vi "online_nonlinear_calibration_save(subVI).vi"(8 "error in (no error)":errorcluster, 9 "Grid Descriptor":cluster{"X Step":sgl, "Y Step":sgl, "Unit":T2}={"X Step"=10.0, "Y Step"=10.0, "Unit"=enum."Millimeter"}, 10 "Image Type":T3 items=["Grayscale (U8)", "Grayscale (I16)", "Grayscale (SGL)", "Complex (CSG)", "RGB (U32)", "HSL (U32)", "RGB (U64)", "Grayscale (U16)"], 11 "Session In":T4="cam0") -> (0 "error out":errorcluster={"status"=TRUE, "code"=-1074396116, "source"="IMAQ CalibrationTargetToPoints\n  "}, 2 "Calibration Axis Info":T5={"Origin Pixel"={"X"=0.0, "Y"=0.0}, "Angle Relative to Horizontal (deg)"=0.0, "X Axis Pixel"={"X"=0.0, "Y"=0.0}, "Axis Reference"=1} {"X Axis Pixel"."Y" format="%.2f"; "X Axis Pixel"."X" format="%.2f"; "Axis Reference" items=["Direct", "Indirect"]; "Angle Relative to Horizontal (deg)" format="%.2f"; "Origin Pixel"."Y" format="%.2f"; "Origin Pixel"."X" format="%.2f"}, 3 "Calibration Template Image Out":T1)   [LabVIEW 2020]
uses:
  <vilib>/vision/Calibration.llb/Error Statistics.ctl
  <vilib>/userDefined/High Color/IMAQdx.ctl
  <vilib>/vision/Image Controls.llb/IMAQ Image.ctl
  <vilib>/vision/Calibration.llb/Distortion Model.ctl
  <vilib>/vision/Calibration.llb/Distortion Model Types.ctl
  <vilib>/vision/NI_Vision_Development_Module.lvlib
panel:
  out "Grey scale image":T1(plugin-control)
  in  "File Path":path=path "D:/desktop/sistemi di visione/foto/calib_info.png"
  out "Error Statistics":T6
  out "Error Map":sgl[][](array[numeric]) format="%.2f"
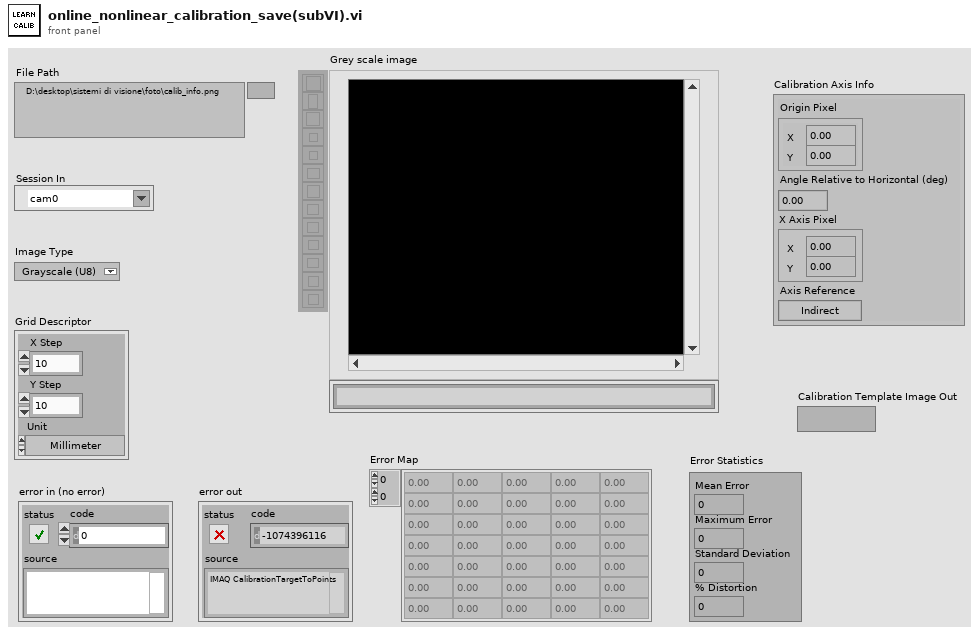
[diagram p1: front panel]
types:
  T1 = typedef "IMAQ Image.ctl" = refnum<image>
  T2 = typedef "Image Unit" = enum32{"Undefined", "Angström", "Micrometer", "Millimeter", "Centimeter", "Meter", "Kilometer", "Microinch", "Inch", "Feet", "Nautical miles", "Standard miles", "Steps"}
  T3 = typedef "Image Type" = u32
  T4 = typedef "IMAQdx.ctl" = refnum<k21>
  T5 = cluster{"Origin Pixel":cluster{"X":sgl, "Y":sgl}, "Angle Relative to Horizontal (deg)":sgl, "X Axis Pixel":cluster{"X":sgl, "Y":sgl}, "Axis Reference":u32}
  T6 = typedef "Error Statistics.ctl" = cluster{"Mean Error":dbl, "Maximum Error":dbl, "Standard Deviation":dbl, "% Distortion":dbl}
  T7 = cluster{"Origin Pixel":cluster{"X":sgl, "Y":sgl}, "Angle Relative to Horizontal (deg)":sgl, "Axis Reference":u32}
  T8 = typedef "Distortion Model.ctl" = cluster{"Distortion Model":T9, "Polynomial Model Setup":cluster{"Radial Coefficient":u32, "Tangential Coefficients ":bool}}
  T9 = typedef "Distortion Model Types.ctl" = i32
  T10 = typedef "Particle Parameters" = i32
  T11 = cluster{"Measurement Parameter":T10, "Range Lower Value":dbl, "Range Upper Value":dbl, "Range":bool, "Measurement Type":bool}[]
  T12 = cluster{"Desired Font (Application)":enum16{"User-specified Font", "Application Font", "System Font", "Dialog Font"}, "[User-specified Font]":cluster{"Font Name":string, "Size":i16, "Strikeout?":bool, "Italic?":bool, "Underline?":bool, "Outline?":bool, "Shadow?":bool, "Bold?":bool, "Rotation Angle":dbl}, "Horizontal Alignment":i16, "Vertical Alignment":i16}
  T13 = typedef "Calibration Reference Points.ctl" = cluster{"Pixel Coordinates":cluster{"X":dbl, "Y":dbl}[], "Real World Coordinates":cluster{"X":dbl, "Y":dbl}[], "Unit":T2, "Image Size":cluster{"X":u32, "Y":u32}}
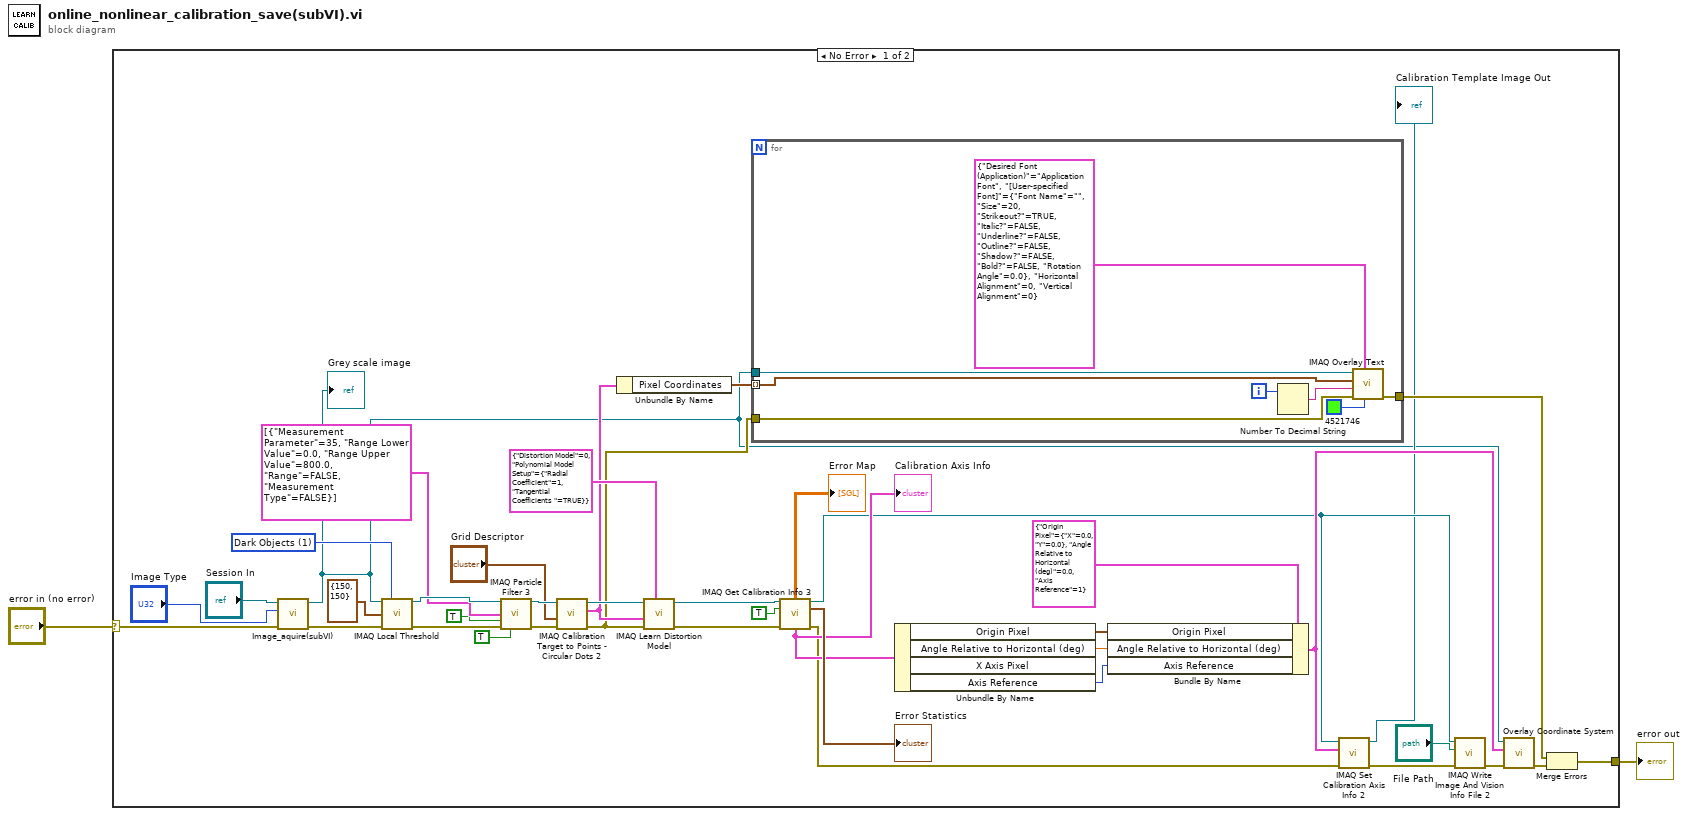
[diagram p0: block diagram]
diagram:
  n1 = case shown="No Error" "error in (no error)" {
    selector: "error in (no error)" -> [w5 w51]
    tunnel: [w22 w51] -> w2
    frame No Error {
      w31 = u32 1 items=["Bright Objects", "Dark Objects"] ("Look For (Bright Objects)")
      n2 = call "Image_aquire(subVI).vi"("error in"=w5, "Image Type"="Image Type", "Session In"="Session In") -> ("error out"=w4:errorcluster, "Grey scale image"=w3:T1)  [unwired: 6 in, 1 out]
      "Grey scale image" <- w3
      n3 = call "IMAQ Local Threshold"("Image Src"=w3, "Look For (Bright Objects)"=w31, "Window Size (32x32)"=cluster{"SizeX":i32, "SizeY":i32} {"SizeX"=150, "SizeY"=150}, "error in (no error)"=w4) -> ("Image Dst Out"=w41:T1, "error out"=w38:errorcluster)  [unwired: 10 in]
      n4 = call "IMAQ Particle Filter 3"("Image Src"=w41, "Selection Values"=T11 [{"Measurement Parameter"=35, "Range Lower Value"=0.0, "Range Upper Value"=800.0, "Range"=FALSE, "Measurement Type"=FALSE}], "Keep/Remove Particles (F)"=TRUE, "error in (no error)"=w38, "Reject Border? (F)"=TRUE) -> ("Image Dst Out"=w39:T1, "error out"=w37:errorcluster)  [unwired: 8 in, 1 out]
      n5 = call "IMAQ Calibration Target to Points - Circular Dots 2"("error in (no error)"=w37, "Grid Descriptor"="Grid Descriptor", "Target Image"=w39) -> ("error out"=w24:errorcluster, "Reference Points"=w25:T13, "Target Image (dup)"=w40:T1)  [unwired: 6 in]
      n6 = Unbundle By Name(w25) -> ("Pixel Coordinates"=w21:cluster{"X":dbl, "Y":dbl}[])
      n7 = call "IMAQ Learn Distortion Model"("Distortion Model Setup"=T8 {"Distortion Model"=0, "Polynomial Model Setup"={"Radial Coefficient"=1, "Tangential Coefficients "=TRUE}}, "error in (no error)"=w24, "Reference Points"=w25, "Calibration Template Image"=w40) -> ("error out"=w36:errorcluster, "Calibration Template Image Out"=w42:T1)  [unwired: 6 in]
      n8 = for {
        tunnel: w24 -> [w50]
        tunnel: [w49] -> w23
        tunnel: w21 -> [w48] mode=indexing
        tunnel: w3 -> [w43]
        i -> [w47]
        n9 = Number To Decimal String(number=w47) -> (decimal integer string=w46:string)  [unwired: 1 in]
        n10 = call "IMAQ Overlay Text"("Text Color (black)"=u32 4521746, "Font, Size & Style"=T12 {"Desired Font (Application)"=enum."Application Font", "[User-specified Font]"={"Font Name"="", "Size"=20, "Strikeout?"=TRUE, "Italic?"=FALSE, "Underline?"=FALSE, "Outline?"=FALSE, "Shadow?"=FALSE, "Bold?"=FALSE, "Rotation Angle"=0.0}, "Horizontal Alignment"=0, "Vertical Alignment"=0}, "error in (no error)"=w50, "String"=w46, "Origin"=w48, "Image"=w43) -> ("error out"=w49:errorcluster)  [unwired: 4 in, 1 out]
      }
      n11 = call "IMAQ Get Calibration Info 3"("Calibration Template Image"=w42, "Return Error Information (False)"=TRUE, "error in (no error)"=w36) -> ("Error Map"=→"Error Map":sgl[][], "Calibration Template Image (duplicate)"=w12:T1, "Error Statistics"=→"Error Statistics":T6, "Calibration Axis Info"=w20:T5, "error out"=w15:errorcluster)  [unwired: 4 in, 4 out]
      "Calibration Axis Info" <- w20
      n12 = Unbundle By Name(w20) -> ("Origin Pixel"=w18:cluster{"X":sgl, "Y":sgl}, "Angle Relative to Horizontal (deg)"=w17:sgl, "Axis Reference"=w16:u32)  [unwired: 1 out]
      n13 = Bundle By Name(cluster=T7 {"Origin Pixel"={"X"=0.0, "Y"=0.0}, "Angle Relative to Horizontal (deg)"=0.0, "Axis Reference"=1} ("Calibration Axis Info 2"), "Origin Pixel"=w18, "Angle Relative to Horizontal (deg)"=w17, "Axis Reference"=w16) -> (w14:T7)
      n14 = call-poly "IMAQ Set Calibration Axis Info 2"("error in (no error)"=w15, "Calibration Axis Info"=w14, "Calibration Template Image In"=w12) -> ("error out"=w11:errorcluster, "Calibration Template Image Out"=→"Calibration Template Image Out":T1)  [unwired: 7 in]
      n15 = call "IMAQ Write Image And Vision Info File 2"("error in (no error)"=w11, "File Path"="File Path", "Image"=w12) -> ("error out"=w10:errorcluster)  [unwired: 7 in, 1 out]
      n16 = call "Overlay Coordinate System.vi"("error in"=w10, "Calibration Axis Info"=w14, "Image"=w3) -> ("error out"=w13:errorcluster)  [unwired: 7 in, 1 out]
      n17 = Merge Errors(w23, w13) -> (w22:errorcluster)
    }
    frame Error {
    }
  }
  "error out" <- w2
